vi "Test Write Complex Number To Serial.vi"() -> ()   [LabVIEW 2014]
uses:
  Complex Numbers.lvlib
panel:
  in  "Error In":errorcluster
  out "Error Out":errorcluster
  out "String complex num.":string
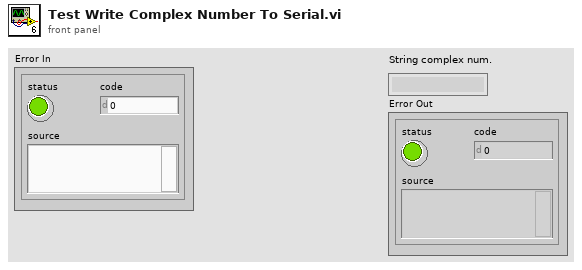
[diagram p1: front panel]
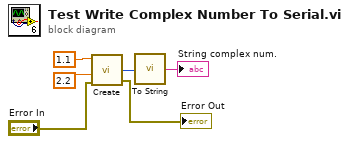
[diagram p0: block diagram]
diagram:
  n1 = call "Create.vi"("Error In"="Error In", "Imag"=2.2, "Real"=1.1) -> ("Error Out"=→"Error Out":errorcluster, "Complex"=w3:u32)  [unwired: 2 in]
  n2 = call "To String.vi"("Complex number"=w3) -> ("String complex num."=→"String complex num.":string)
